vi "Start.vi"(8 "error in (no error)":errorcluster, 11 "TestBlock in":refnum<class "TestBlock.lvclass">) -> (0 "error out":errorcluster, 3 "TestBlock out":refnum<class "TestBlock.lvclass">)   [LabVIEW 2020, in "TestBlock.lvclass"]
uses:
  TestBlock.lvclass
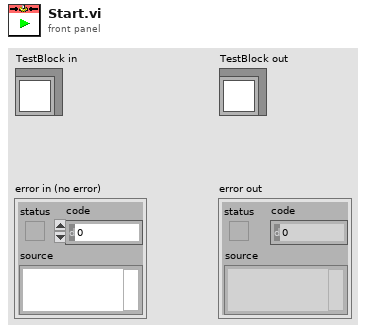
[diagram p1: front panel]
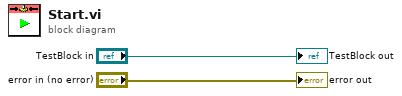
[diagram p0: block diagram]
diagram:
  "error out" <- "error in (no error)"
  "TestBlock out" <- "TestBlock in"
